vi "Actor Core.vi"(8 "error in":errorcluster, 11 "MockModel in":refnum<class "MockModelOneShotPublish.lvclass">) -> (0 "error out":errorcluster, 3 "Actor out":refnum<class "Actor.lvclass">)   [LabVIEW 2015, in "MockModel.lvlib" / "MockModelOneShotPublish.lvclass"]
doc: "(<B>Filename</B>: Actor Framework.lvlib:Actor.lvclass:Actor Core.vi)\n\nReceives messages to the actor, reacts to them, and initiates any error handling that may shut the actor down.\n\nDescendant classes may override this VI to append parallel tasks for the actor to complete while it handles messages. Overrides use the Call Parent Method node."
uses:
  MockModelOneShotPublish.lvclass
  <vilib>/ActorFramework/Actor/Actor.lvclass
  Framework/IModel/IModel/IModel.lvclass/IModel.ctl
  Framework/AbstractMessages/PreAddressedMsg/PreAddressedMsg.lvclass/PreAddressedMsg.ctl
  Framework/IMediator/IMediator Messages/Publish Msg/Publish Msg.lvclass/Publish Msg.ctl
  <vilib>/ActorFramework/Message Enqueuer/Message Enqueuer.lvclass/Message Enqueuer.ctl
  Framework/IMediator/IMediator Messages/Publish Msg/Send Pre-Addressed Publish.vi
  <vilib>/ActorFramework/Message Enqueuer/Enqueue.vi
  Framework/AbstractMessages/PreAddressedMsg/Read Return Address.vi
  <vilib>/ActorFramework/Message Priority Queue/Priority Enqueue.vi
  Framework/IModel/IModel/IModel.lvclass
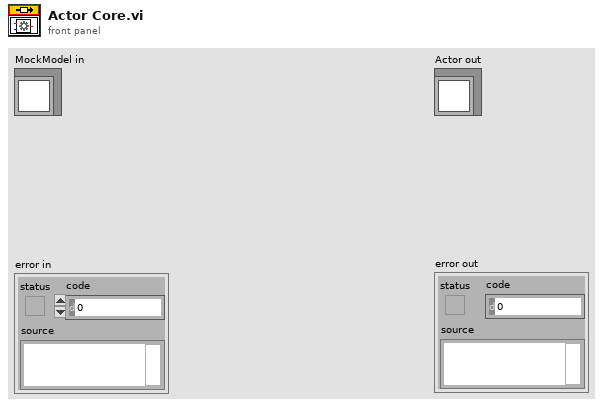
[diagram p1: front panel]
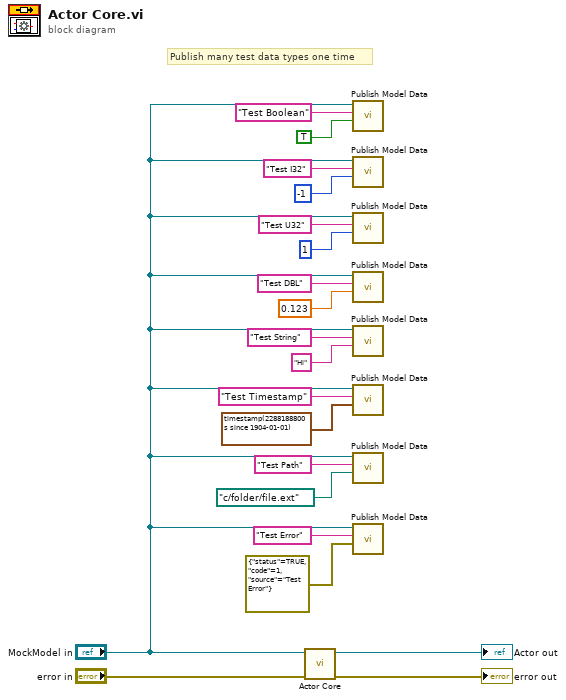
[diagram p0: block diagram]
diagram:
  # "Publish many test data types one time"
  n1 = call-parent "Actor Core.vi"("error in"="error in", "Actor in"="MockModel in") -> ("error out"=→"error out":errorcluster, "Actor out"=→"Actor out":refnum<class "Actor.lvclass">)  [unwired: 8 in]
  n2 = call "Publish Model Data.vi"("Data to Publish"=TRUE, "Topic Name"="Test Boolean", "IModel in"="MockModel in") -> ()  [unwired: 7 in, 2 out]
  n3 = call "Publish Model Data.vi"("Data to Publish"=-1 ("Topic Name"), "Topic Name"="Test I32", "IModel in"="MockModel in") -> ()  [unwired: 7 in, 2 out]
  n4 = call "Publish Model Data.vi"("Data to Publish"=u32 1 ("Topic Name"), "Topic Name"="Test U32", "IModel in"="MockModel in") -> ()  [unwired: 7 in, 2 out]
  n5 = call "Publish Model Data.vi"("Data to Publish"=0.123 ("Topic Name"), "Topic Name"="Test DBL", "IModel in"="MockModel in") -> ()  [unwired: 7 in, 2 out]
  n6 = call "Publish Model Data.vi"("Data to Publish"="Hi" ("Topic Name"), "Topic Name"="Test String", "IModel in"="MockModel in") -> ()  [unwired: 7 in, 2 out]
  n7 = call "Publish Model Data.vi"("Data to Publish"=timestamp(2288188800 s since 1904-01-01) ("Topic Name"), "Topic Name"="Test Timestamp", "IModel in"="MockModel in") -> ()  [unwired: 7 in, 2 out]
  n8 = call "Publish Model Data.vi"("Data to Publish"=path "c:/folder/file.ext" ("Topic Name"), "Topic Name"="Test Path", "IModel in"="MockModel in") -> ()  [unwired: 7 in, 2 out]
  n9 = call "Publish Model Data.vi"("Data to Publish"=errorcluster {"status"=TRUE, "code"=1, "source"="Test Error"} ("Topic Name"), "Topic Name"="Test Error", "IModel in"="MockModel in") -> ()  [unwired: 7 in, 2 out]
